vi "mongo_c_wrapper_test.vi"() -> ()   [LabVIEW 2013]
panel:
  out "error out":errorcluster
  out "outer loops":i32
  out "inner loops":i32
  out "key":string
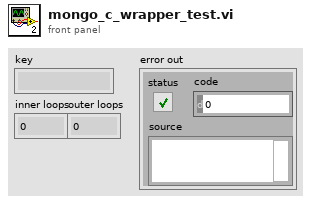
[diagram p1: front panel]
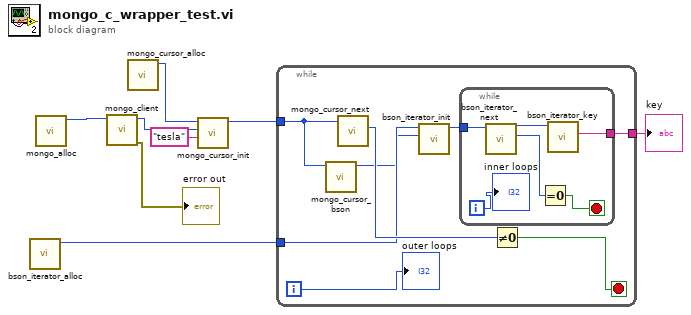
[diagram p0: block diagram]
diagram:
  n1 = call "bson_iterator_alloc.vi"() -> ("bson_iterator ptr"=w3:u32)  [unwired: 11 in]
  n2 = call "mongo_alloc.vi"() -> ("mongo pointer"=w8:u32)  [unwired: 11 in]
  n3 = call "mongo_client.vi"("conn ptr in"=w8) -> ("error out"=→"error out":errorcluster, "conn ptr out"=w6:u32)  [unwired: 8 in, 1 out]
  n4 = call "mongo_cursor_alloc.vi"() -> ("mongo_cursor ptr"=w7:u32)  [unwired: 11 in]
  n5 = call "mongo_cursor_init.vi"("ns"="tesla", "conn ptr"=w6, "cursor ptr"=w7) -> ("cursor ptr out"=w4:u32)  [unwired: 7 in, 1 out]
  n6 = while {
    tunnel: w4 -> [w12]
    tunnel: w3 -> [w14]
    tunnel: [w10] -> w2
    i -> [w9]
    stop <- w15 stop-if-true
    n7 = call "mongo_cursor_bson.vi"("cursor ptr"=w12) -> ("bson ptr"=w13:u32)  [unwired: 10 in]
    n8 = call "mongo_cursor_next.vi"("cursor ptr"=w12) -> ("return type"=w16:i32)  [unwired: 9 in, 1 out]
    n9 = call "bson_iterator_init.vi"("bson ptr"=w13, "bson_iterator ptr"=w14) -> ("bson_iterator ptr out"=w11:u32)  [unwired: 8 in, 1 out]
    n10 = while {
      tunnel: w11 -> [w22]
      tunnel: [w18] -> w10
      i -> [w17]
      stop <- w21 stop-if-true
      n11 = call "bson_iterator_next.vi"("bson_iterator ptr"=w22) -> ("returned bson_type"=w20:i32, "bson_iterator ptr out"=w19:u32)  [unwired: 9 in]
      n12 = Equal To 0?(x=w20) -> (x = 0?=w21:bool)
      n13 = call "bson_iterator_key.vi"("bson_iterator ptr"=w19) -> ("key"=w18:string)  [unwired: 9 in, 1 out]
      "inner loops" <- w17
    }
    n14 = Not Equal To 0?(x=w16) -> (x != 0?=w15:bool)
    "outer loops" <- w9
  }
  "key" <- w2
